vi "CSM - Message Console.vi"() -> ()   [LabVIEW 2017]
doc: "CSM Debug Console, you can use this tool:\n\n1. Select an existing CSM instance, open the front panel and block diagram.\n2. Scan the API interfaces of existing CSM instances.\n3. Select an API interface, call synchronously or asynchronously, view the return value.\n4. View the overall program's running log."
uses:
  _Support/Typedef/_CSM_GlobalLog_MSG.ctl
  _Support/Typedef/_CSM_Response Source Message.ctl
  _Support/Typedef/_CSM_GlobalLog_MSG_TYPE.ctl
  _jksm/_action.ctl
  1437127e-efa5-494e-aa43-da9d647a7a6f.vi
  6c6a0a0d-4e90-432b-9646-7a8ac0ceadb8.vi
  <vilib>/addons/_JKI Toolkits/State Machine/_JKI_lib_State_Machine.llb/Parse State Queue__JKI_lib_State_Machine.vi
  AdvanceAPI/CSM - Convert Error to Argument.vi
  _Support/GlobalEvent/GEvt-Generate with Rule Check.vi
  AdvanceAPI/CSM - Keywords.vi
  _Support/GlobalEvent/Cache-GEvt Refs.vi
  _Support/GlobalEvent/LogFilter/LogFilter - Check.vi
  <vilib>/Utility/Data Type/Get Type Information.vi
  _csmHelper/lvcsmFile/lvcsm File Path.vi
  <vilib>/Utility/config.llb/Open Config Data.vi
  <vilib>/Utility/config.llb/Read Key.vi
  <vilib>/Utility/config.llb/Read Key (Boolean).vi
  <vilib>/Utility/config.llb/Read Key (String).vi
  <vilib>/Utility/Data Type/Get Array Information.vi
  <vilib>/Utility/config.llb/Get Key Names.vi
  _csmHelper/lvcsmFile/Path to lvcsm String.vi
  _csmHelper/lvcsmFile/lvcsm String to Path.vi
  <vilib>/Utility/config.llb/Read Key (I32).vi
  <vilib>/Utility/config.llb/Read Key (Double).vi
  <vilib>/Utility/config.llb/Close Config Data.vi
  _csmHelper/lvcsmFile/_Array of VData to VCluster.vi
  <vilib>/Utility/config.llb/Write Key.vi
  <vilib>/Utility/config.llb/Write Key (Boolean).vi
  <vilib>/Utility/config.llb/Remove Key.vi
  <vilib>/Utility/config.llb/Write Key (String).vi
  <vilib>/Utility/config.llb/Write Key (I32).vi
  <vilib>/Utility/config.llb/Write Key (Double).vi
  _Polymophic/Build Synchronous Message with Arguments.vi
  _Polymophic/Build No-Reply Asynchronous Message with Arguments.vi
  _Polymophic/Build Interrupt Broadcast Message.vi
  _Support/GlobalEvent/LogFilter/LogFilter.lvclass
  Communicable State Machine.lvlib
  _csmHelper/API with lvcsm Support/CSM-Helper API with lvcsm Support.lvlib
  _csmHelper/CSM-Helper.lvclass
  _Shared/CSM Shared.lvlib
  _ui/csm-ui-support.lvlib
  _jksm/_jkism_magic.lvlib
panel:
  in  "Timeout(s)":i32=10 caption="(s)" min=1 max=180 step=1 format="%.0p"
  in  "Interface-Filter":enum16{"API-Only", "UserDef States", "All"}(ring)
  in  "Refresh API":bool
  in  "MsgString":string(combo)
  in  "Sync (-@)":bool
  in  "Async (->|)":bool
  in  "CSM":string
  in  "Arguments":string
  in  "Revert Safe String":bool=TRUE
  out "Response":string
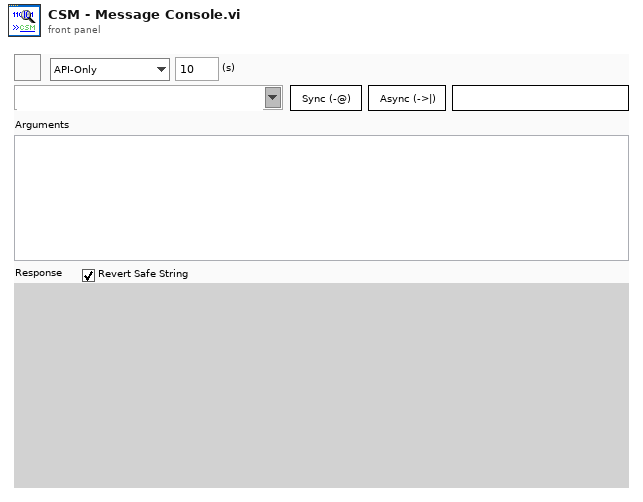
[diagram p1: front panel]
types:
  T1 = enum32{"Invalid", "Standard", "Closed", "Hidden", "Minimized", "Maximized"}
  T2 = enum32{"invalid app kind", "Development System", "Run Time System", "Student Edition", "Embedded LabVIEW", "Evaluation", "Custom"}
  T3 = cluster{"Response Timeout(s)":i32, "History Length":i32, "History":string[], "Periodic Enable":bool, "Periodic threashold(#/s)":dbl, "Periodic Check Peroid(s)":dbl}
  T4 = typedef "_jkism_magic.lvlib/_action.ctl" = enum16{"Obtain", "Destroy", "Broadcast", "Post"}
  T5 = cluster{"Shift":bool, "Ctrl":bool, "Alt":bool, "Cmd":bool, "Opt":bool}
  T6 = cluster{"Core":cluster{"Current VI Reference":refnum<vi>, "Close Panel on Exit?":bool}, "CSM Global Log Event":refnum<user-event>, "Toobar.advance":refnum<vi>[], "CSM Check History":string[], "History Length":i32}
  T7 = cluster{"Current VI Reference":refnum<vi>, "Close Panel on Exit?":bool}
  T8 = enum8{"Enabled", "Disabled", "Disabled and Grayed Out"}
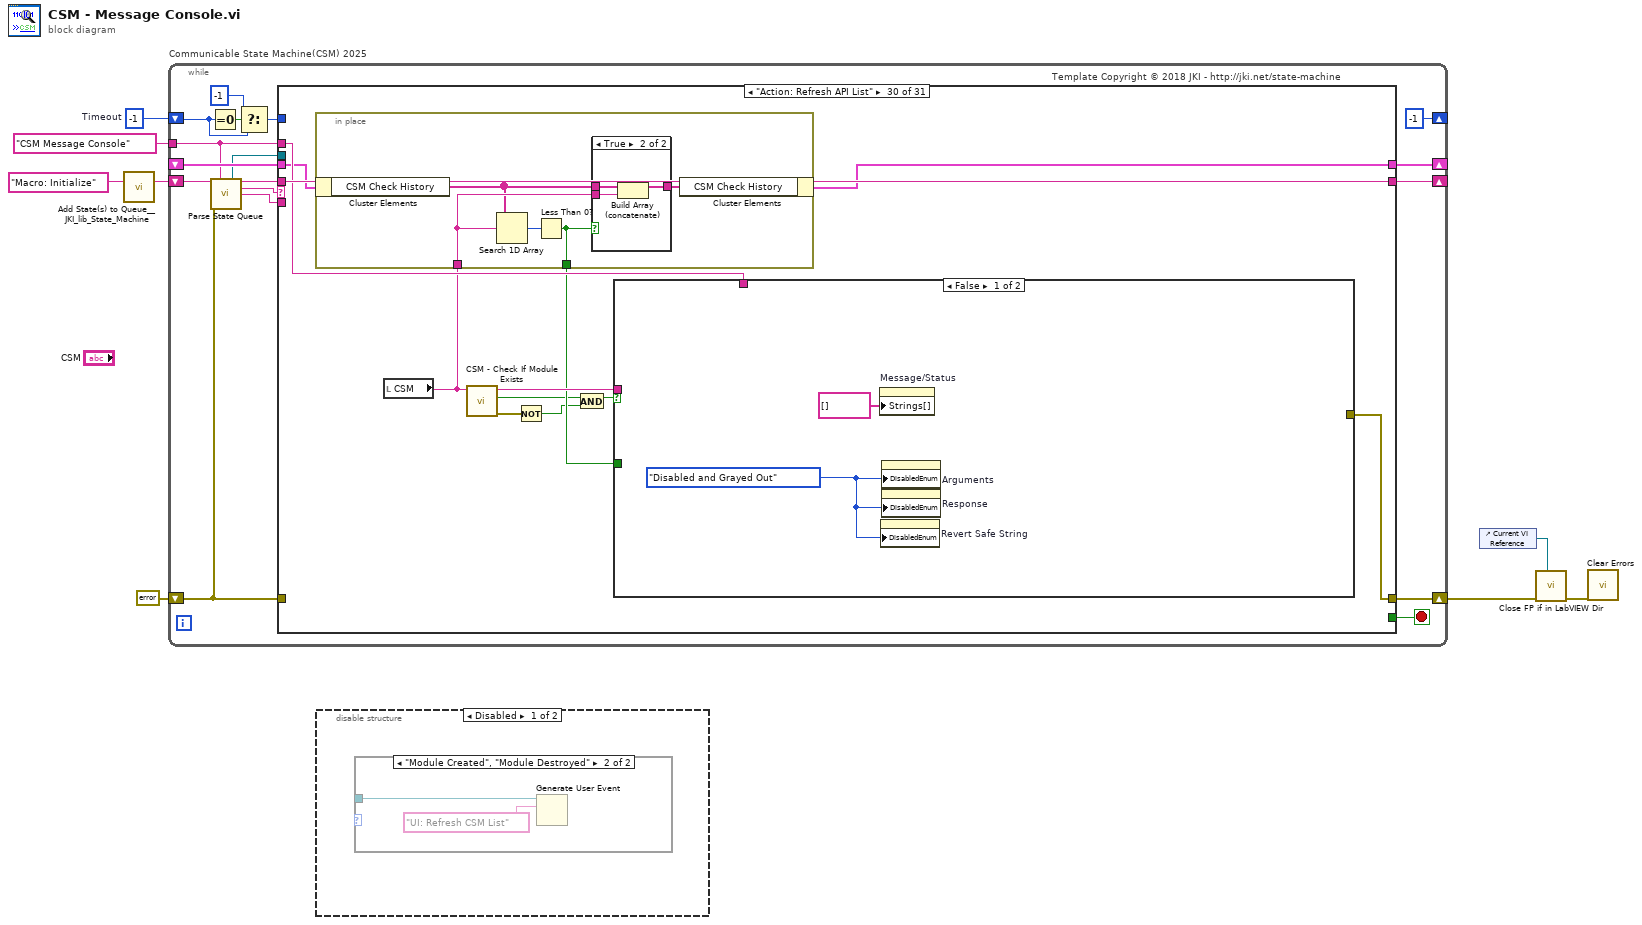
[diagram p0: block diagram]
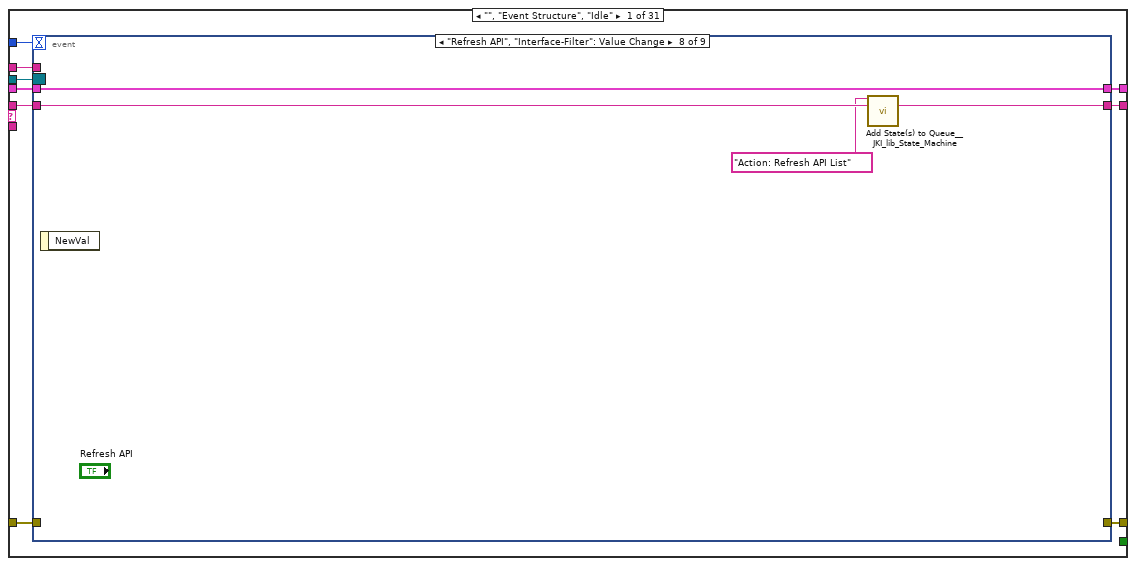
[diagram p4: hidden frame]
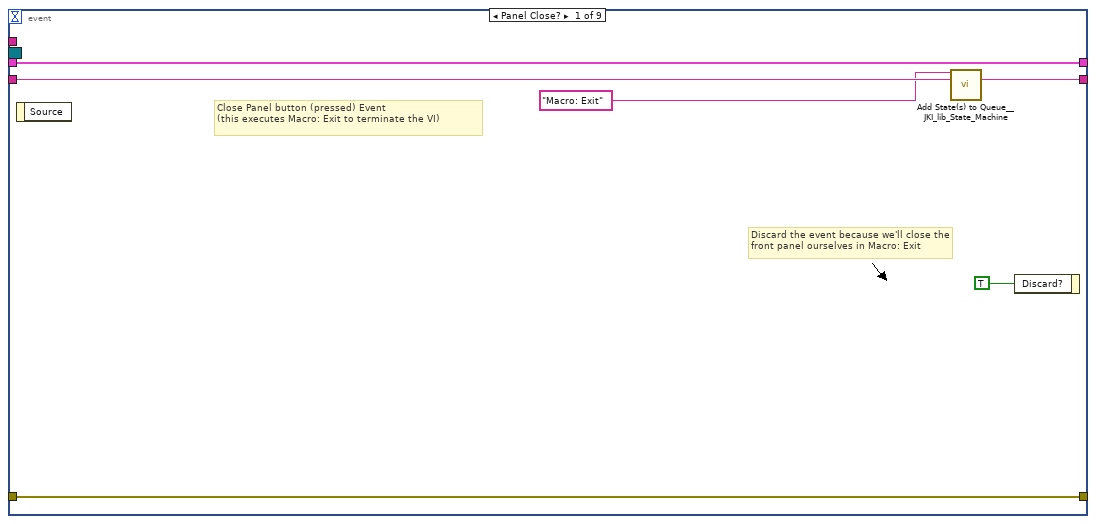
[diagram p5: hidden frame]
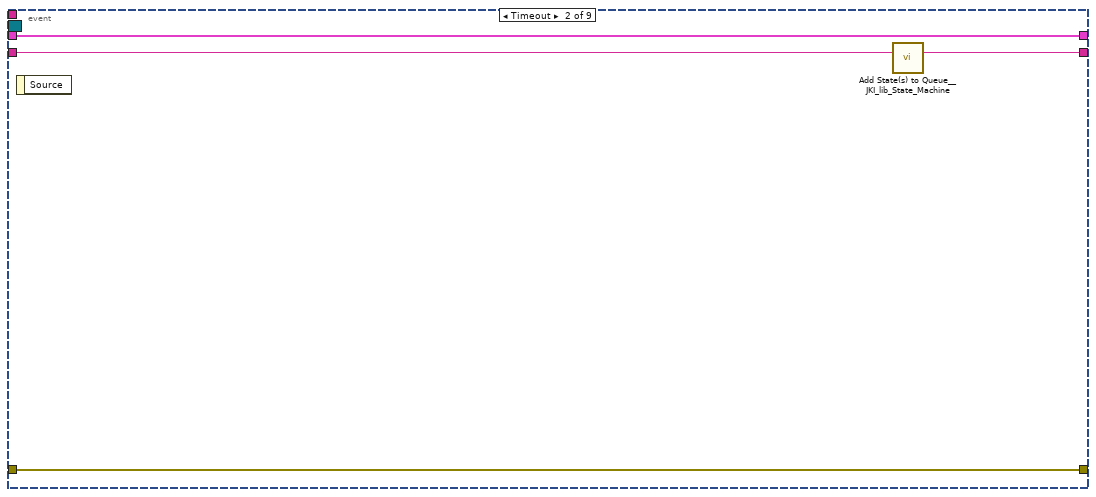
[diagram p6: hidden frame]
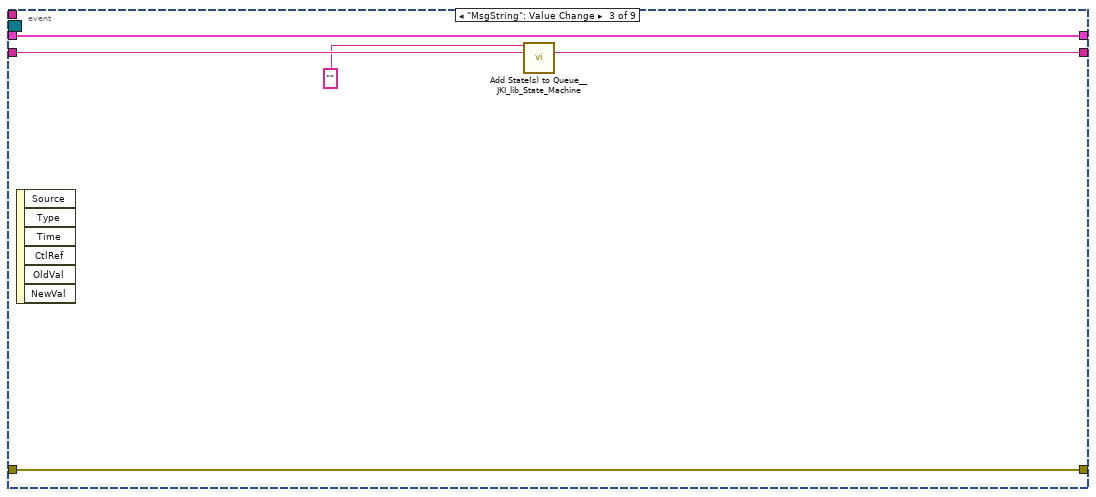
[diagram p7: hidden frame]
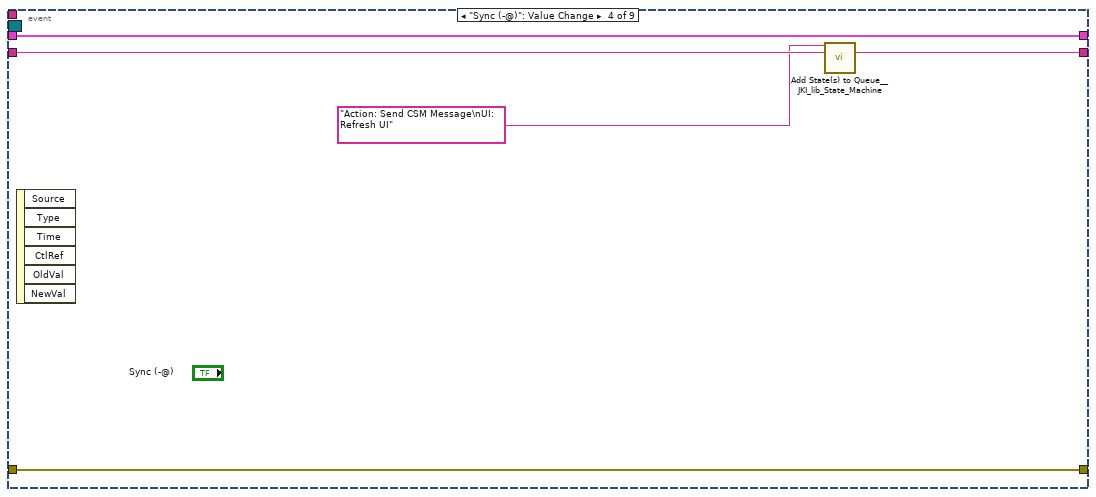
[diagram p8: hidden frame]
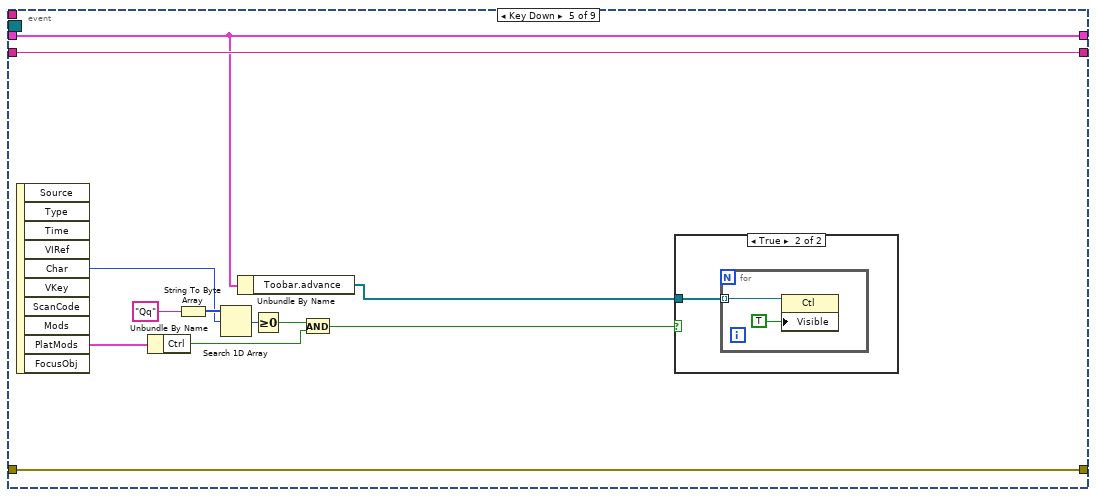
[diagram p9: hidden frame]
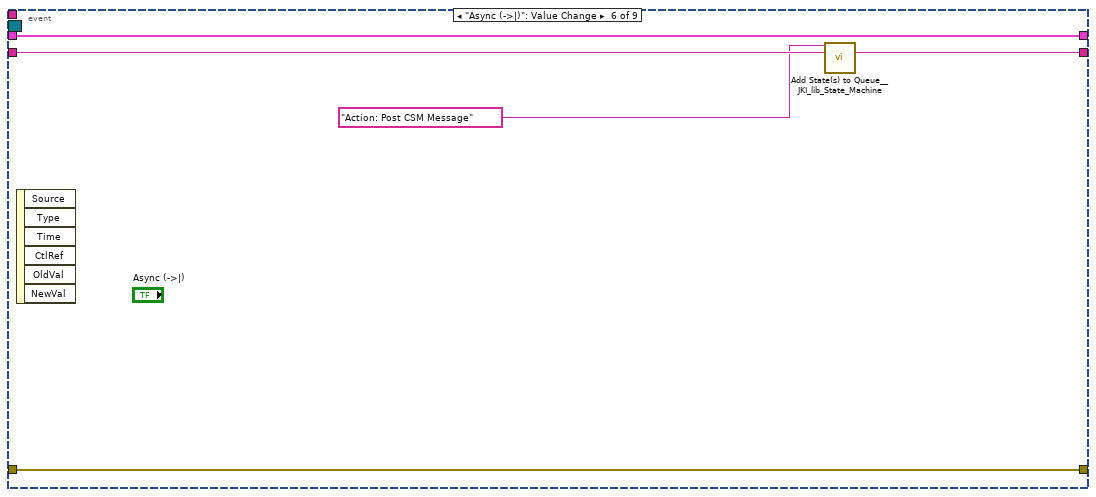
[diagram p11: hidden frame]
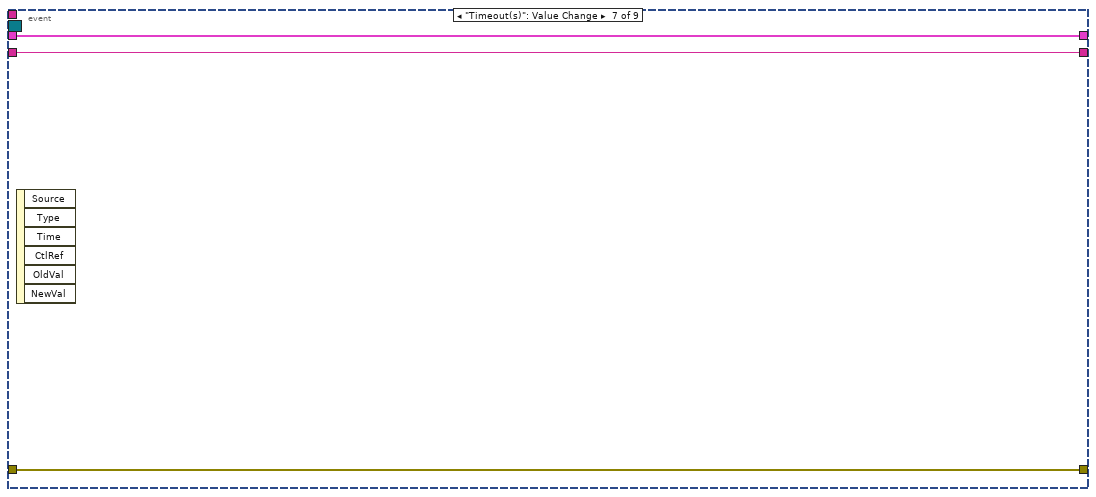
[diagram p12: hidden frame]
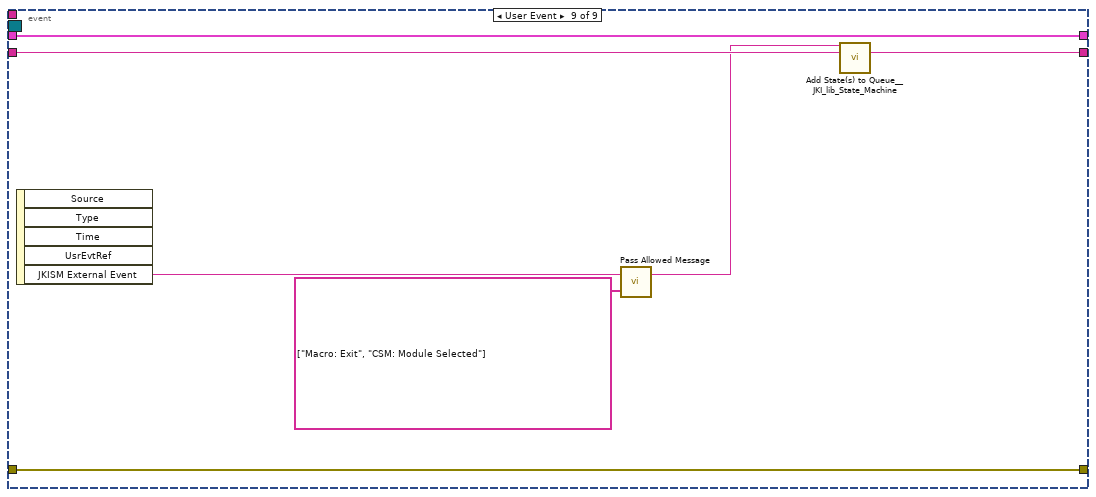
[diagram p13: hidden frame]
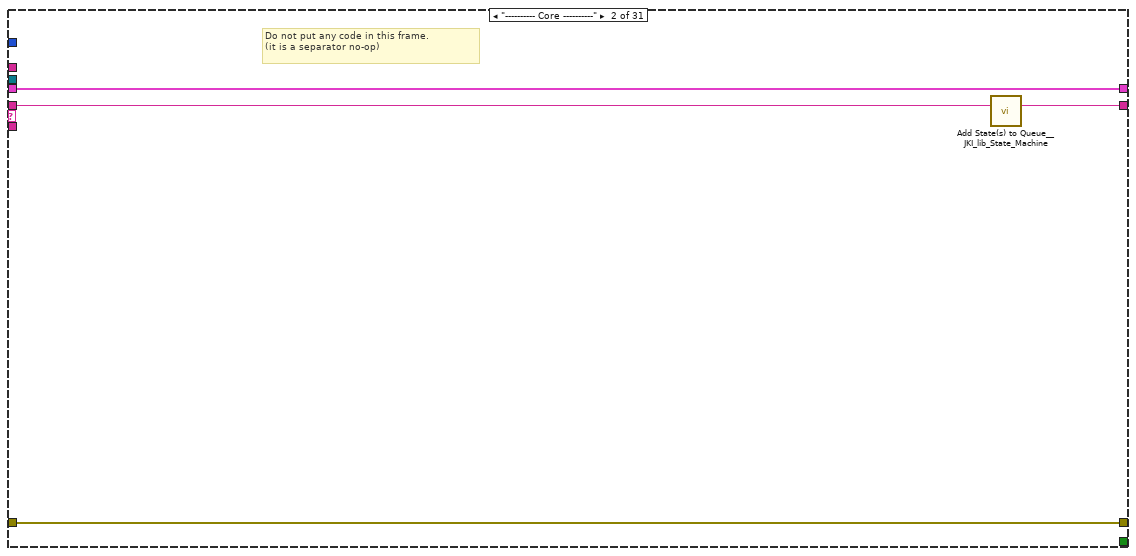
[diagram p14: hidden frame]
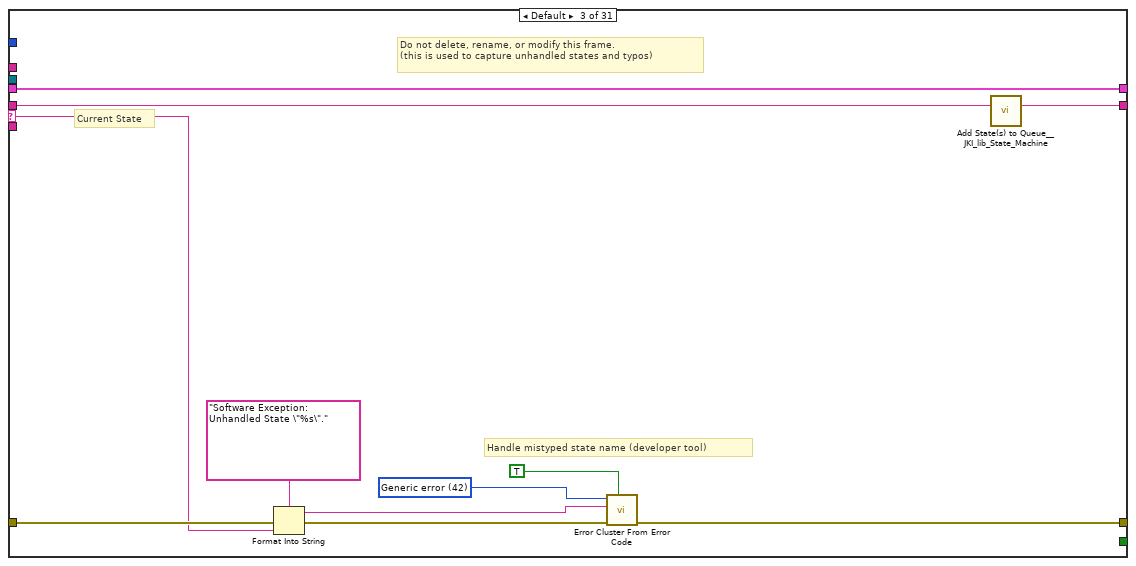
[diagram p15: hidden frame]
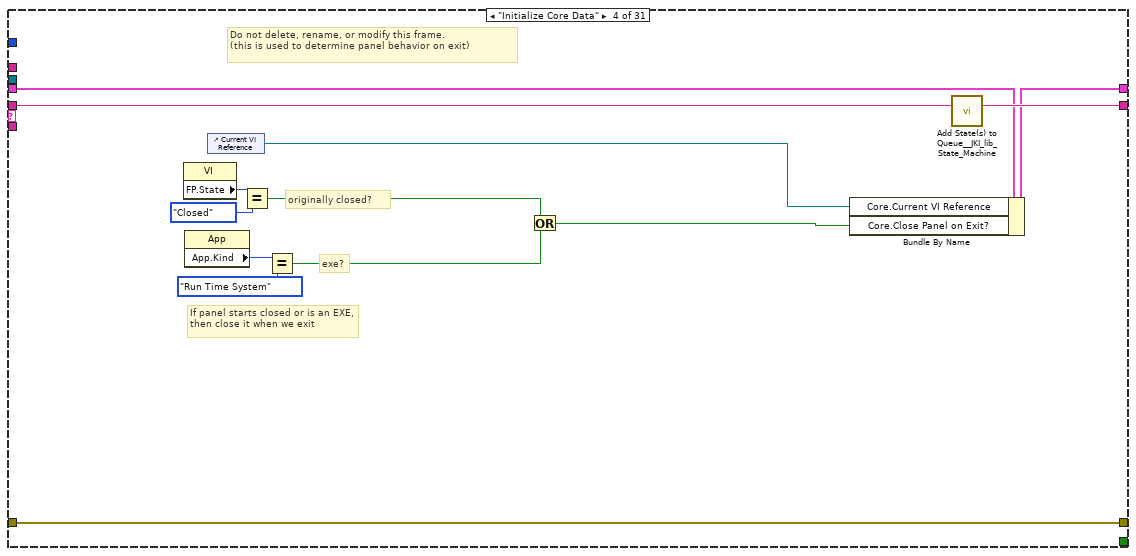
[diagram p16: hidden frame]
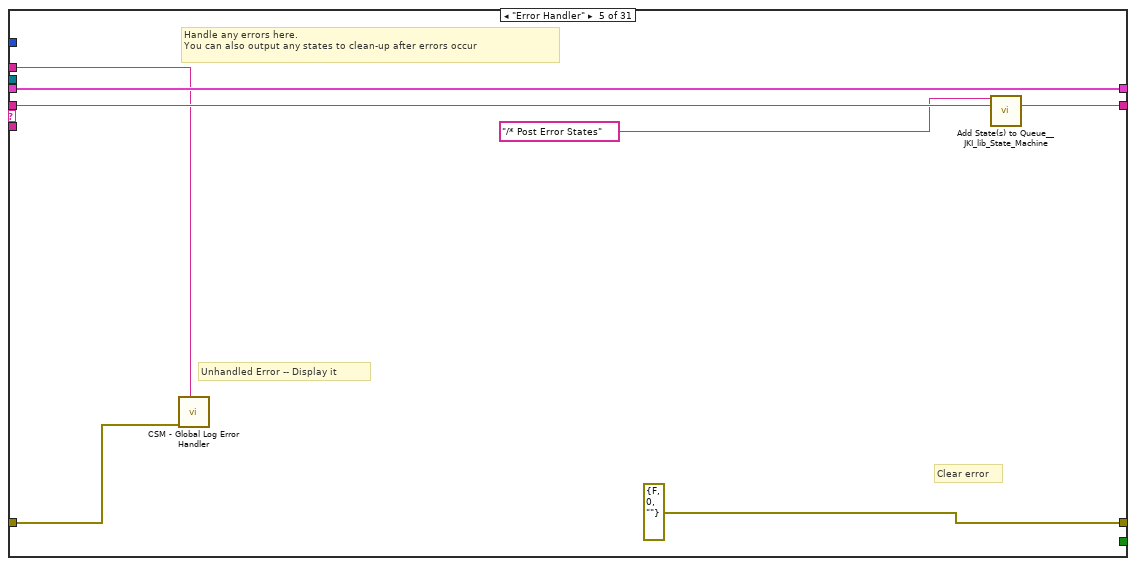
[diagram p17: hidden frame]
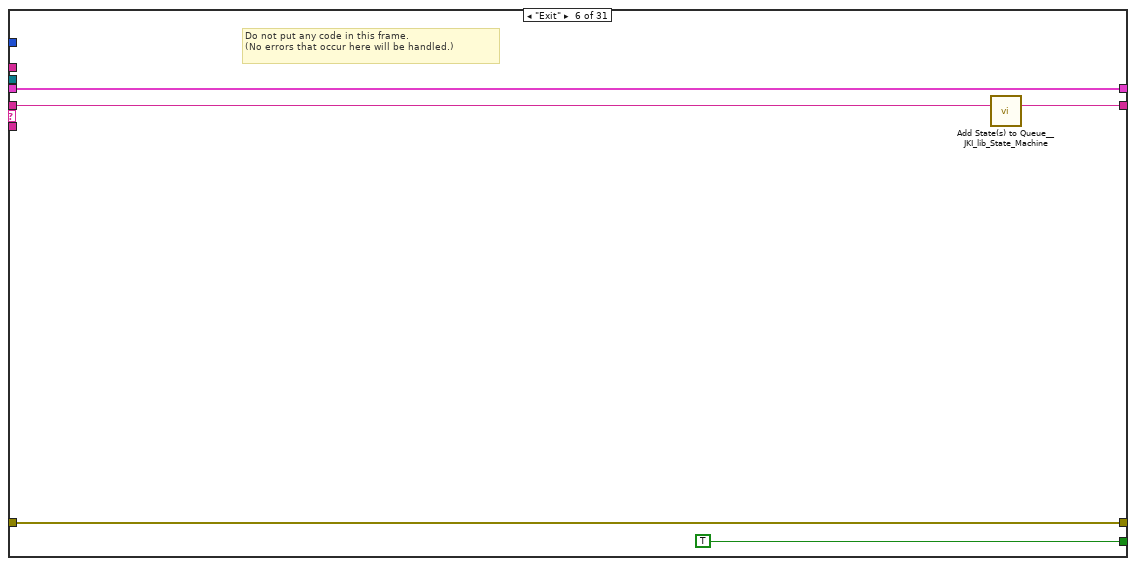
[diagram p18: hidden frame]
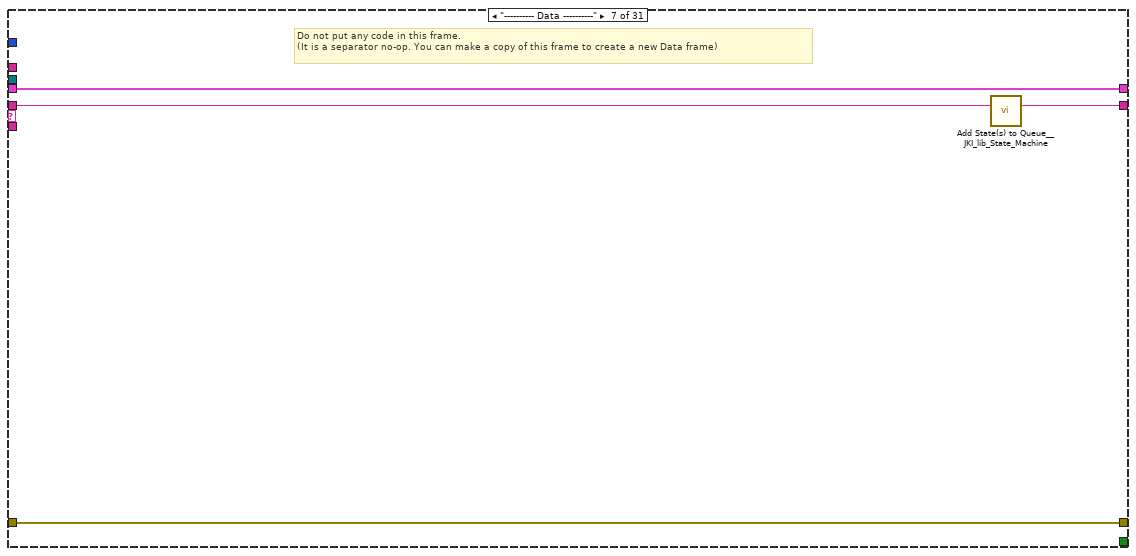
[diagram p19: hidden frame]
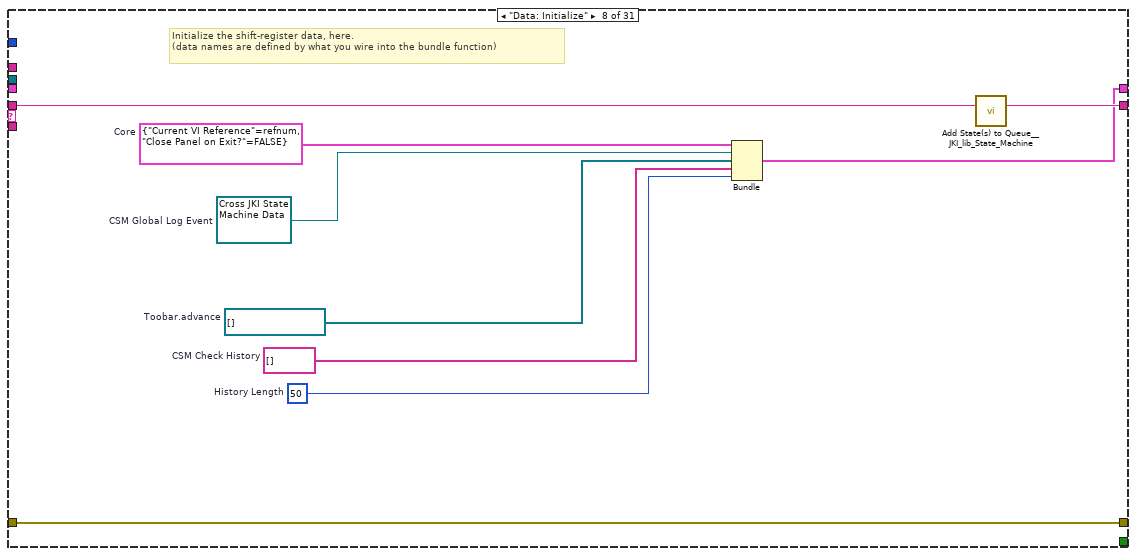
[diagram p20: hidden frame]
diagram:
  w6 = -1  # Timeout
  n1 = call <vilib>:"Add State(s) to Queue__JKI_lib_State_Machine.vi"("State(s) in (\"\")"="Macro: Initialize") -> ("States Out"=w7:string)  [unwired: 14 in]
  n2 = while "Communicable State Machine(CSM) 2025" {
    shift-right: [w18] -> _
    shift-left: _ -> [w17]
    shift-right: [w21] -> w3
    shift-left: errorcluster {"status"=FALSE, "code"=0, "source"=""} ("error out") -> [w16]
    shift-right: [w20] -> _
    shift-left: w7 -> [w22]
    tunnel: "CSM Message Console" -> [w10]
    shift-right: [-1 ("Timeout")] -> _
    shift-left: w6 -> [w13]
    stop <- w19 stop-if-true
    # "Template Copyright © 2018 JKI - http://jki.net/state-machine"
    n3 = Equal To 0?(x=w13) -> (x = 0?=w15:bool)
    n4 = call "Parse State Queue.vi"("State Queue"=w22, "Current Module(\"\" to generate an ID)"=w10, "Error In (no error)"=w16) -> ("Event Registration Refnum"=w9:refnum<event-registration>, "Remaining States"=w24:string, "Current State"=w25:string, "Arguments"=w23:string)  [unwired: 9 in]
    n5 = Select(t=-1 ("Timeout"), s=w15, f=w13) -> (s? t:f=w12:i32)
    n6 = case shown="\"Action: Refresh API List\"" w25 {
      selector: w25 -> [_ _ w93 _ _ _ _ _ _ _ _ _ _ _ _ _ _ _ _ _ _ _ _ _ _ _ _ _ _ _ _]
      tunnel: w24 -> [w34 w92 w97 w116 w123 w128 w132 w141 w143 w152 w160 w166 w170 w174 w181 w190 w201 w276 w283 w286 w292 w297 w302 w310 w314 w325 w350 w369 w383 w396 w424]
      tunnel: w23 -> [_ _ _ _ _ _ _ _ _ _ _ _ _ _ _ w185 w195 w275 _ w288 _ _ _ _ _ _ _ _ _ _ _]
      tunnel: w17 -> [w32 w89 w95 w109 w120 w126 w129 _ w142 w150 w159 w161 w167 w171 w178 w188 w197 w273 w282 w289 w291 w294 w299 w307 w311 w323 w348 w367 w382 w391 w423]
      tunnel: [w31 w90 w99 w113 errorcluster {"status"=FALSE, "code"=0, "source"=""} ("error out") w125 w130 w138 w144 _ w155 w162 w168 w172 w179 w186 w198 w277 w284 w290 w293 w295 w300 w308 w312 w320 w347 w366 w384 w393 w425] -> w21
      tunnel: w16 -> [w30 w90 w98 w113 w119 w125 w130 w138 w144 _ _ w163 w168 w172 w179 w187 w199 w277 w284 w290 w293 w295 w300 w308 w312 _ _ _ w384 _ w425]
      tunnel: [w33 w91 w96 w115 w122 w127 w131 w140 w143 w152 w160 w165 w169 w173 w180 w189 w200 w276 w283 w287 w292 w296 w301 w309 w313 w324 w349 w368 w383 w396 w424] -> w20
      tunnel: [_ _ _ _ _ TRUE _ _ _ _ _ _ _ _ _ _ _ _ _ _ _ _ _ _ _ _ _ _ _ _ _] -> w19
      tunnel: [w29 w89 w95 w114 w120 w126 w129 w139 w142 w151 w159 w161 w167 w171 w178 w188 w197 w273 w282 w289 w291 w294 w299 w307 w311 w323 w348 w367 w382 w390 w423] -> w18
      tunnel: w12 -> [w28 _ _ _ _ _ _ _ _ _ _ _ _ _ _ _ _ _ _ _ _ _ _ _ _ _ _ _ _ _ _]
      tunnel: w10 -> [w27 _ _ _ w117 _ _ _ _ w147 w156 _ _ _ _ _ _ _ _ _ _ _ _ _ _ _ _ _ _ w394 _]
      tunnel: w9 -> [w26 _ _ _ _ _ _ _ _ _ _ _ _ _ _ _ _ _ _ _ _ _ _ _ _ _ _ _ _ _ _]
      frame "", "Event Structure", "Idle" {
        n7 = event shown="[7] \"Refresh API\", \"Interface-Filter\": Value Change" {
          selector: w26 -> [_ _ _ _ _ _ _ _ _]
          dyn-events: _ -> [_ _ _ _ _ _ _ _ _]
          timeout: w28 -> [_ _ _ _ _ _ _ _ _]
          tunnel: w34 -> [w40 w44 w46 w51 w66 w71 w77 w79 w85]
          tunnel: [w39 w43 w47 w52 w66 w72 w77 w80 w86] -> w33
          tunnel: w32 -> [w37 w41 w48 w53 w55 w73 w75 w81 w87]
          tunnel: [w38 w42 w49 w54 w65 w74 w76 _ w88] -> w31
          tunnel: w30 -> [w38 w42 w49 w54 w65 w74 w76 _ w88]
          tunnel: [w37 w41 w48 w53 w55 w73 w75 w81 w87] -> w29
          tunnel: w27 -> [_ _ _ _ _ _ _ _ _]
          event Panel Close? {
            # "Discard the event because we'll close the front panel ourselves in Macro: Exit"
            # "Close Panel button (pressed) Event\n(this executes Macro: Exit to terminate the VI)"
            n8 = event-data() -> ()  [unwired: 1 in, 1 out]
            n9 = call <vilib>:"Add State(s) to Queue__JKI_lib_State_Machine.vi"("State(s) in Front (\"\")"="Macro: Exit", "State(s) in (\"\")"=w40) -> ("States Out"=w39:string)  [unwired: 13 in]
            n10 = event-data("Discard?"=TRUE) -> ()  [unwired: 1 in, 1 out]
          }
          event Timeout {
            n11 = event-data() -> ()  [unwired: 1 in, 1 out]
            n12 = call <vilib>:"Add State(s) to Queue__JKI_lib_State_Machine.vi"("State(s) in (\"\")"=w44) -> ("States Out"=w43:string)  [unwired: 14 in]
          }
          event "MsgString": Value Change {
            n13 = event-data() -> ()  [unwired: 1 in, 6 out]
            n14 = call <vilib>:"Add State(s) to Queue__JKI_lib_State_Machine.vi"("State(s) in Front (\"\")"="" ("State(s) in Front (\"\")"), "State(s) in (\"\")"=w46) -> ("States Out"=w47:string)  [unwired: 13 in]
          }
          event "Sync (-@)": Value Change {
            n15 = event-data() -> ()  [unwired: 1 in, 6 out]
            n16 = call <vilib>:"Add State(s) to Queue__JKI_lib_State_Machine.vi"("State(s) in Front (\"\")"="Action: Send CSM Message\nUI: Refresh UI" ("State(s) in Front (\"\")"), "State(s) in (\"\")"=w51) -> ("States Out"=w52:string)  [unwired: 13 in]
          }
          event Key Down {
            n17 = event-data() -> ("Char"=w56:i16, "PlatMods"=w57:T5)  [unwired: 1 in, 8 out]
            n18 = Unbundle By Name(w57) -> ("Ctrl"=w60:bool)
            n19 = String To Byte Array(string="Qq") -> (unsigned byte array=w62:u8[])
            n20 = Search 1D Array(1D array=w62, element=w56) -> (index of element=w63:i32)  [unwired: 1 in]
            n21 = Unbundle By Name(w55) -> ("Toobar.advance"=w58:refnum<vi>[])
            n22 = Greater Or Equal To 0?(x=w63) -> (x >= 0?=w64:bool)
            n23 = And(x=w64, y=w60) -> (x .and. y?=w59:bool)
            n24 = case shown="True" w59 {
              tunnel: w58 -> [_ w67]
              frame False {
              }
              frame True {
                n25 = for {
                  tunnel: w67 -> [w69] mode=indexing
                  n26 = property class="Ctl"(reference=w69, "Visible"=TRUE) -> ()  [unwired: 1 in, 2 out]
                }
              }
            }
          }
          event "Async (->|)": Value Change {
            n27 = event-data() -> ()  [unwired: 1 in, 6 out]
            n28 = call <vilib>:"Add State(s) to Queue__JKI_lib_State_Machine.vi"("State(s) in Front (\"\")"="Action: Post CSM Message" ("State(s) in Front (\"\")"), "State(s) in (\"\")"=w71) -> ("States Out"=w72:string)  [unwired: 13 in]
          }
          event "Timeout(s)": Value Change {
            n29 = event-data() -> ()  [unwired: 1 in, 6 out]
          }
          event "Refresh API", "Interface-Filter": Value Change {
            n30 = event-data() -> ()  [unwired: 1 in, 1 out]
            n31 = call <vilib>:"Add State(s) to Queue__JKI_lib_State_Machine.vi"("State(s) in Front (\"\")"="Action: Refresh API List" ("State(s) in Front (\"\")"), "State(s) in (\"\")"=w79) -> ("States Out"=w80:string)  [unwired: 13 in]
          }
          event User Event {
            n32 = event-data() -> ("JKISM External Event"=w84:string)  [unwired: 1 in, 4 out]
            n33 = call "Pass Allowed Message.vi"("Allowed Message"=string[] ["Macro: Exit", "CSM: Module Selected"], "JKISM External Event"=w84) -> ("States"=w83:string)  [unwired: 1 in]
            n34 = call <vilib>:"Add State(s) to Queue__JKI_lib_State_Machine.vi"("State(s) in Front (\"\")"=w83, "State(s) in (\"\")"=w85) -> ("States Out"=w86:string)  [unwired: 13 in]
          }
        }
      }
      frame "---------- Core ----------" {
        # "Do not put any code in this frame.\n(it is a separator no-op)"
        n35 = call <vilib>:"Add State(s) to Queue__JKI_lib_State_Machine.vi"("State(s) in (\"\")"=w92) -> ("States Out"=w91:string)  [unwired: 14 in]
      }
      frame Default {
        w102 = 42 items=["No error", "Argument error", "Memory is full", "Out of zone", "End of file", "File already open", "Generic file I/O error", "File not found", "File permission error", "Disk is full", "Duplicate path", "Too many files open", "System feature not enabled", "Resource file not found", "Cannot add resource", "Resource not found", "Image not found", "Image memory error", "Pen does not exist", "Config type invalid", "Config token not found", "Config parse error", "Config memory error", "Bad external code format", "Bad external code offset", "External code not present", "Null window", "Destroy window error", "Null menu", "Print aborted", "Bad print record", "Print driver error", "Windows error during printing", "Memory error during printing", "Print dialog error", "Generic print error", "Invalid device refnum", "Device not found", "Device parameter error", "Device unit error", "Cannot open device", "Device call aborted", "Generic error", "Cancelled by user", "Object ID too low", "Object ID too high", "Object not in heap", "Unknown heap", "Unknown object (invalid DefProc)", "Unknown object (DefProc not in table)", "Message out of range", "Invalid (null) method", "Unknown message", "Manager call not supported", "Bad address", "Network operation in progress", "Network operation timed out", "Connection is busy", "Network attribute not supported", "Network error", "Address in use", "System out of memory", "Connection aborted", "Connection refused", "Not connected", "Already connected", "Connection closed", "Initialization error (interapplication manager)", "Bad occurrence", "Wait on unbound occurrence handler", "Occurrence queue overflow", "Datalog type conflict", "Unused", "Unrecognized type (interapplication manager)", "Memory corrupt", "Failed to make temporary DLL", "Old CIN version", "Drag socket not found", "Failed to load drop-object", "Failed to register OLE object", "Failed to release OLE object", "Format specifier type mismatch", "Unknown format specifier", "Too few format specifiers", "Too many format specifiers", "Scan failed", "Newer CIN version", "Error converting to variant", "Runtime menu error", "Password tampered", "Variant attribute not found", "Incompatible variant data type", "Event data is not available", "Event Store is not present", "Occurrence is not found", "Event Queue is not created", "Event info is not available", "Refnum passed is NULL", "Error retrieving Class GUID", "Error retrieving CoClass GUID", "Error retrieving TypeLib GUID.", "Bad built application magic bytes.", "Specific driver is different from the specific driver associated with the Logical Name.", "There is no session opened to the class driver.", "Max Error", "MAX - Error with config objects", "MAX - Error loading configuration", "MAX - Group not supported"]
        # "Current State"
        # "Do not delete, rename, or modify this frame.\n(this is used to capture unhandled states and typos)"
        # "Handle mistyped state name (developer tool)"
        n36 = Format Into String(format string="Software Exception: Unhandled State \"%s\"." ("message"), error in=w98, w93) -> (resulting string=w101:string, error out=w100:errorcluster)  [unwired: 1 in]
        n37 = call <vilib>:"Error Cluster From Error Code.vi"("show call chain? (False)"=TRUE, "error in (no error)"=w100, "error message (\"\")"=w101, "error code (0)"=w102) -> ("error out"=w99:errorcluster)  [unwired: 5 in]
        n38 = call <vilib>:"Add State(s) to Queue__JKI_lib_State_Machine.vi"("State(s) in (\"\")"=w97) -> ("States Out"=w96:string)  [unwired: 14 in]
      }
      frame "Initialize Core Data" {
        # "Do not delete, rename, or modify this frame.\n(this is used to determine panel behavior on exit)"
        # "originally closed?"
        # "exe?"
        # "If panel starts closed or is an EXE, then close it when we exit"
        n39 = property class="VI"() -> ("FP.State"=w106:T1)  [unwired: 2 in, 2 out]
        n40 = property class="App"() -> ("App.Kind"=w112:T2)  [unwired: 2 in, 2 out]
        n41 = control-ref of="Current VI Reference"() -> (w107:refnum<vi>)
        n42 = Equal?(x=w106, y=T1."Closed" ("Front Panel Window:State")) -> (x = y?=w104:bool)
        n43 = Equal?(x=w112, y=T2."Run Time System" ("Application:Kind")) -> (x = y?=w110:bool)
        n44 = Or(x=w104, y=w110) -> (x .or. y?=w108:bool)
        n45 = Bundle By Name(cluster=w109, "Core.Current VI Reference"=w107, "Core.Close Panel on Exit?"=w108) -> (w114:T6)
        n46 = call <vilib>:"Add State(s) to Queue__JKI_lib_State_Machine.vi"("State(s) in (\"\")"=w116) -> ("States Out"=w115:string)  [unwired: 14 in]
      }
      frame "Error Handler" {
        # "Unhandled Error -- Display it"
        # "Handle any errors here.\nYou can also output any states to clean-up after errors occur"
        # "Clear error"
        n47 = call "CSM - Global Log Error Handler.vi"("Place (\"\" to Use VI's Name)"=w117, "Error In"=w119) -> ()  [unwired: 9 in, 1 out]
        n48 = call <vilib>:"Add State(s) to Queue__JKI_lib_State_Machine.vi"("State(s) in Front (\"\")"="/* Post Error States", "State(s) in (\"\")"=w123) -> ("States Out"=w122:string)  [unwired: 13 in]
      }
      frame "Exit" {
        # "Do not put any code in this frame.\n(No errors that occur here will be handled.)"
        n49 = call <vilib>:"Add State(s) to Queue__JKI_lib_State_Machine.vi"("State(s) in (\"\")"=w128) -> ("States Out"=w127:string)  [unwired: 14 in]
      }
      frame "---------- Data ----------" {
        # "Do not put any code in this frame.\n(It is a separator no-op. You can make a copy of this frame to create a new Data frame)"
        n50 = call <vilib>:"Add State(s) to Queue__JKI_lib_State_Machine.vi"("State(s) in (\"\")"=w132) -> ("States Out"=w131:string)  [unwired: 14 in]
      }
      frame "Data: Initialize" {
        w133 = 50  # History Length
        w134 = string[] []  # CSM Check History
        w135 = refnum<vi>[] []  # Toobar.advance
        w136 = refnum<user-event> refnum  # CSM Global Log Event
        w137 = T7 {"Current VI Reference"=refnum, "Close Panel on Exit?"=FALSE}  # Core
        # "Initialize the shift-register data, here.\n(data names are defined by what you wire into the bundle function)"
        n51 = Bundle("Core"=w137, "CSM Global Log Event"=w136, "Toobar.advance"=w135, "CSM Check History"=w134, "History Length"=w133) -> (w139:T6)  [unwired: 1 in]
        n52 = call <vilib>:"Add State(s) to Queue__JKI_lib_State_Machine.vi"("State(s) in (\"\")"=w141) -> ("States Out"=w140:string)  [unwired: 14 in]
      }
      frame "Data: Initialize References" {
      }
      frame "Data: Load Arguments Config File" {
        n53 = call "lvcsm Read Cluster.vim"("Section"=w147, "Default Prototype"=T3 {"Response Timeout(s)"=30, "History Length"=50, "History"=[], "Periodic Enable"=TRUE, "Periodic threashold(#/s)"=0.5, "Periodic Check Peroid(s)"=3.0}) -> ("Cluster (Dup)"=w149:T3)  [unwired: 8 in, 1 out]
        n54 = Unbundle By Name(w149) -> ("Response Timeout(s)"=w148:i32, "History Length"=w145:i32)  [unwired: 4 out]
        n55 = local write "Timeout(s)"(w148) -> ()
        n56 = Bundle By Name(cluster=w150, "History Length"=w145) -> (w151:T6)
      }
      frame "Data: Save Arguments Config File" {
        n57 = Unbundle By Name(w159) -> ("History Length"=w153:i32)
        n58 = local read "Timeout(s)"() -> (w157:i32)
        n59 = Bundle By Name(cluster=T3 {"Response Timeout(s)"=30, "History Length"=50, "History"=[], "Periodic Enable"=TRUE, "Periodic threashold(#/s)"=0.5, "Periodic Check Peroid(s)"=3.0}, "Response Timeout(s)"=w157, "History Length"=w153) -> (w158:T3)
        n60 = call "lvcsm Write Cluster.vim"("Section"=w156, "Configuration"=w158) -> ("error out"=w155:errorcluster)  [unwired: 9 in]
      }
      frame "Data: Cleanup" {
        # "Cleanup any data and references, here.\n(this is called automatically, by the Macro: Exit)"
        n61 = Unbundle By Name(w161) -> ("Core.Current VI Reference"=w164:refnum<vi>)
        n62 = Close Reference(reference=w164, error in (no error)=w163) -> (error out=w162:errorcluster)
        n63 = call <vilib>:"Add State(s) to Queue__JKI_lib_State_Machine.vi"("State(s) in (\"\")"=w166) -> ("States Out"=w165:string)  [unwired: 14 in]
      }
      frame "---------- Events ----------" {
        # "Do not put any code in this frame.\n(It is a separator no-op. You can make a copy of this frame to create a new UI frame)"
        n64 = call <vilib>:"Add State(s) to Queue__JKI_lib_State_Machine.vi"("State(s) in (\"\")"=w170) -> ("States Out"=w169:string)  [unwired: 14 in]
      }
      frame "---------- UI ----------" {
        # "Do not put any code in this frame.\n(It is a separator no-op. You can make a copy of this frame to create a new UI frame)"
        n65 = call <vilib>:"Add State(s) to Queue__JKI_lib_State_Machine.vi"("State(s) in (\"\")"=w174) -> ("States Out"=w173:string)  [unwired: 14 in]
      }
      frame "UI: Initialize" {
        # "Initialize the User Interface, here.\n(this is called automatically, by the Macro: Init)"
        n66 = Unbundle By Name(w178) -> ("Toobar.advance"=w177:refnum<vi>[])
        n67 = disable-structure shown="Disabled" {
          disable-tunnel: w177 -> [w182 _]
          frame Disabled {
            n68 = for {
              tunnel: w182 -> [w184] mode=indexing
              n69 = property class="Ctl"(reference=w184, "Visible"=FALSE) -> ()  [unwired: 1 in, 2 out]
            }
          }
          frame Enabled {
          }
        }
        n70 = local write "Response"(" " ("State History")) -> ()
        n71 = local write "Interface-Filter"(enum16{"API-Only", "UserDef States", "All"}."UserDef States" ("Interface-Filter")) -> ()
        n72 = call <vilib>:"Add State(s) to Queue__JKI_lib_State_Machine.vi"("State(s) in (\"\")"=w181) -> ("States Out"=w180:string)  [unwired: 14 in]
      }
      frame "UI: Cursor Set" {
        # "Argument"
        # "Set and Unset Cursor Busy.\n(Usage: \"UI: Cursor Set >> Busy|Idle\")"
        n73 = case shown="\"Idle\", Default" w185 {
          tunnel: w187 -> [w192 w194]
          tunnel: [w191 w193] -> w186
          frame "Idle", Default {
            n74 = call <vilib>:"Unset Busy.vi"("error in (no error)"=w192) -> ("error out"=w191:errorcluster)  [unwired: 10 in]
          }
          frame "Busy" {
            n75 = call <vilib>:"Set Busy.vi"("error in (no error)"=w194) -> ("error out"=w193:errorcluster)  [unwired: 9 in, 1 out]
          }
        }
        n76 = call <vilib>:"Add State(s) to Queue__JKI_lib_State_Machine.vi"("State(s) in (\"\")"=w190) -> ("States Out"=w189:string)  [unwired: 14 in]
      }
      frame "UI: Front Panel State" {
        # "Argument"
        # "Set Front Panel Open or Closed\n(Usage: \"UI: Front Panel State >> Open|Close\")"
        n77 = Unbundle By Name(w197) -> ("Core.Current VI Reference"=w196:refnum<vi>)
        n78 = case shown="\"Minimize\", \"Minimized\"" w195 {
          tunnel: w199 -> [w207 w222 w233 w246 w259]
          tunnel: [w209 w223 w235 w248 w261] -> w198
          tunnel: w196 -> [w208 w220 w234 w247 w260]
          frame "Open", "Standard", Default {
            w202 = T1."Standard" ("State")
            n79 = property class="VI"(reference=w208, error in=w207) -> (reference out=w205:refnum<vi>, error out=w206:errorcluster, "FP.State"=w204:T1)
            n80 = Not Equal?(x=w204, y=w202) -> (x != y?=w203:bool)
            n81 = case shown="True" w203 {
              tunnel: [w213 w215] -> w209
              tunnel: w206 -> [w212 w215]
              tunnel: w205 -> [w211 _]
              tunnel: w202 -> [w210 _]
              frame True {
                n82 = invoke class="VI" method="FP.Open"(reference=w211, error in=w212, "Activate"=TRUE, "State"=w210) -> (error out=w213:errorcluster)  [unwired: 1 in, 4 out]
              }
              frame False {
              }
            }
          }
          frame "Close", "Closed" {
            n83 = property class="VI"(reference=w220, error in=w222) -> (reference out=w219:refnum<vi>, error out=w221:errorcluster, "FP.State"=w217:T1)
            n84 = Not Equal?(x=w217, y=T1."Closed" ("Front Panel Window:State")) -> (x != y?=w216:bool)
            n85 = case shown="True" w216 {
              tunnel: [w224 w227] -> w223
              tunnel: w221 -> [w224 w226]
              tunnel: w219 -> [_ w225]
              frame False {
              }
              frame True {
                n86 = invoke class="VI" method="FP.Close"(reference=w225, error in=w226) -> (error out=w227:errorcluster)  [unwired: 1 in, 2 out]
              }
            }
          }
          frame "Hidden", "Hide" {
            w228 = T1."Hidden" ("State")
            n87 = property class="VI"(reference=w234, error in=w233) -> (reference out=w231:refnum<vi>, error out=w232:errorcluster, "FP.State"=w230:T1)
            n88 = Not Equal?(x=w230, y=w228) -> (x != y?=w229:bool)
            n89 = case shown="True" w229 {
              tunnel: [w239 w240] -> w235
              tunnel: w232 -> [w238 w240]
              tunnel: w231 -> [w237 _]
              tunnel: w228 -> [w236 _]
              frame True {
                n90 = invoke class="VI" method="FP.Open"(reference=w237, error in=w238, "State"=w236) -> (error out=w239:errorcluster)  [unwired: 2 in, 4 out]
              }
              frame False {
              }
            }
          }
          frame "Minimize", "Minimized" {
            w241 = T1."Minimized" ("State")
            n91 = property class="VI"(reference=w247, error in=w246) -> (reference out=w244:refnum<vi>, error out=w245:errorcluster, "FP.State"=w243:T1)
            n92 = Not Equal?(x=w243, y=w241) -> (x != y?=w242:bool)
            n93 = case shown="True" w242 {
              tunnel: [w252 w253] -> w248
              tunnel: w245 -> [w251 w253]
              tunnel: w244 -> [w250 _]
              tunnel: w241 -> [w249 _]
              frame True {
                n94 = invoke class="VI" method="FP.Open"(reference=w250, error in=w251, "State"=w249) -> (error out=w252:errorcluster)  [unwired: 2 in, 4 out]
              }
              frame False {
              }
            }
          }
          frame "Maximize", "Maximized" {
            w254 = T1."Maximized" ("State")
            n95 = property class="VI"(reference=w260, error in=w259) -> (reference out=w257:refnum<vi>, error out=w258:errorcluster, "FP.State"=w256:T1)
            n96 = Not Equal?(x=w256, y=w254) -> (x != y?=w255:bool)
            n97 = case shown="True" w255 {
              tunnel: [w265 w266] -> w261
              tunnel: w258 -> [w264 w266]
              tunnel: w257 -> [w263 _]
              tunnel: w254 -> [w262 _]
              frame True {
                n98 = invoke class="VI" method="FP.Open"(reference=w263, error in=w264, "State"=w262) -> (error out=w265:errorcluster)  [unwired: 2 in, 4 out]
              }
              frame False {
              }
            }
          }
        }
        n99 = call <vilib>:"Add State(s) to Queue__JKI_lib_State_Machine.vi"("State(s) in (\"\")"=w201) -> ("States Out"=w200:string)  [unwired: 14 in]
      }
      frame "UI: Autoset Arguments" {
        n100 = call "CSM - Revert Arguments-Safe String.vi"("Safe Argument String"=w275) -> ("Origin Argument String"=w267:string)  [unwired: 8 in]
        n101 = control-ref of="CSM"() -> (w270:refnum<vi>)
        n102 = call "Remove Comments from Single-line.vi"("single-line text"=w267) -> ("single-line text without comments"=w274:string)  [unwired: 2 in]
        n103 = call "Split Single-line Message.vi"("single-line text"=w274) -> ("state"=w272:string, "args"=w271:string, "source/target"=w269:string)  [unwired: 6 in, 1 out]
        n104 = case shown="\"<interrupt>\", \"<status>\"" w269 {
          selector: w269 -> [w278 _]
          tunnel: [w278 w279] -> w268
          tunnel: w267 -> [_ w280]
          frame Default {
            (unwired) enum32{"Message", "Status"}."Message" ("Tab(Msg/Status)")
          }
          frame "<interrupt>", "<status>" {
            (unwired) enum32{"Message", "Status"}."Status" ("Tab(Msg/Status)")
            n105 = Match Pattern(string=w280, regular expression="//") -> (after substring=w279:string)  [unwired: 1 in, 3 out]
          }
        }
        n106 = local write "MsgString"(w272) -> ()
        n107 = local write "Arguments"(w271) -> ()
        n108 = property on="Property Node" class="Str"(reference=w270, "Value"=w268) -> ()  [unwired: 1 in, 2 out]
      }
      frame "UI: Refresh History List" {
      }
      frame "CSM: Module Selected" {
        n109 = local write "CSM"(w288) -> ()
        n110 = call <vilib>:"Add State(s) to Queue__jki_lib_state_machine.vi"("State(s) in Front (\"\")"="Action: Refresh API List" ("State(s) in Front (\"\")"), "State(s) in (\"\")"=w286) -> ("States Out"=w287:string)  [unwired: 13 in]
      }
      frame "UI: Refresh UI" {
      }
      frame "---------- Macro ----------" {
        # "Do not put any code in this frame.\n(It is a separator no-op. You can make a copy of this frame to create a new Macro frame)"
        n111 = call <vilib>:"Add State(s) to Queue__JKI_lib_State_Machine.vi"("State(s) in (\"\")"=w297) -> ("States Out"=w296:string)  [unwired: 14 in]
      }
      frame "Macro: Initialize" {
        # "Initialization Macro\n(This is called once, when the VI starts)"
        n112 = call <vilib>:"Add State(s) to Queue__JKI_lib_State_Machine.vi"("State(s) in Front (\"\")"="Data: Initialize\nData: Initialize References\nInitialize Core Data\nUI: Initialize\nData: Load Arguments Config File\nUI: Front Panel State >> Open\nAction: Refresh API List\nAction: Change Btn States", "State(s) in (\"\")"=w302) -> ("States Out"=w301:string)  [unwired: 13 in]
      }
      frame "Macro: Exit" {
        # "Exit Macro\n(This is called once, when the VI exits)"
        n113 = call "FGV-JKISM Modules.vi"("Enum"=_action."Broadcast", "Message"="Macro: Exit") -> ()  [unwired: 8 in, 2 out]
        n114 = call <vilib>:"Add State(s) to Queue__JKI_lib_State_Machine.vi"("State(s) at Back (\"\")"="Data: Save Arguments Config File\nData: Cleanup\nExit") -> ("States Out"=w305:string)  [unwired: 14 in]
        n115 = call <vilib>:"Add State(s) to Queue__JKI_lib_State_Machine.vi"("State(s) in Front (\"\")"=w305, "State(s) in (\"\")"=w310) -> ("States Out"=w309:string)  [unwired: 13 in]
      }
      frame "---------- Action ----------" {
        # "Template Separator\n(You can make a copy of, or modify, this frame)"
        n116 = call <vilib>:"Add State(s) to Queue__JKI_lib_State_Machine.vi"("State(s) in (\"\")"=w314) -> ("States Out"=w313:string)  [unwired: 14 in]
      }
      frame "Action: Send CSM Message" {
        n117 = local read "CSM"() -> (w319:string)
        n118 = Multiply(x=1000, y="Timeout(s)") -> (x*y=w316:i32)
        n119 = case shown="\"\"" "MsgString" {
          selector: "MsgString" -> [_ w332]
          tunnel: "Arguments" -> [_ w331]
          tunnel: [_ w337] -> w320
          tunnel: w319 -> [_ w330]
          tunnel: [_ w329] -> w318
          tunnel: w316 -> [_ w336]
          frame "" {
          }
          frame Default {
            n120 = call "CSM - Send Message and Wait for Reply.vi"("Response Timeout (-2 Using Global Settings)"=w336, "Current Module (\"\" to Generate an ID)"="Tool-Testpnl" ("Current Module(\"\" to generate an ID)"), "Target Module"=w330, "Arguments (\"\")"=w331, "State"=w332) -> ("error out"=w337:errorcluster, "Response"=w339:string)  [unwired: 4 in, 1 out]
            n121 = call-poly "Build Message with Arguments++.vi"("State With Arguments"=w332, "Arguments (\"\")"=w331, "Target Module (\"\")"=w330) -> ("CSM Message String"=w334:string)  [unwired: 12 in]
            n122 = case shown="True" "Revert Safe String" {
              tunnel: w339 -> [w340 w342]
              tunnel: [w340 w341] -> w327
              frame False {
              }
              frame True {
                n123 = call "CSM - Revert Arguments-Safe String.vi"("Safe Argument String"=w342) -> ("Origin Argument String"=w341:string)  [unwired: 8 in]
              }
            }
            "Response" <- w327
            n124 = call "CSM - Make String Arguments Safe.vi"("Argument String"=w334) -> ("Safe Argument String"=w333:string)  [unwired: 8 in]
            n125 = call <vilib>:"Build State String with Arguments__JKI_lib_State_Machine.vi"("Arguments (\"\")"=w333, "State"="" ("State(s) in Front (\"\")")) -> ("State with Arguments"=w328:string)  [unwired: 4 in]
            n126 = call <vilib>:"Add State(s) to Queue__JKI_lib_State_Machine.vi"("State(s) in (\"\")"=w328) -> ("States Out"=w329:string)  [unwired: 14 in]
          }
        }
        n127 = call <vilib>:"Add State(s) to Queue__JKI_lib_State_Machine.vi"("State(s) in (\"\")"=w325, "State(s) at Back (\"\")"=w318) -> ("States Out"=w324:string)  [unwired: 13 in]
      }
      frame "Action: Post CSM Message" {
        # "Your code here.\n(You can make a copy of, or modify, this frame)"
        n128 = local read "MsgString"() -> (w343:string)
        n129 = local read "Arguments"() -> (w344:string)
        n130 = local read "CSM"() -> (w346:string)
        n131 = case shown="Default" w343 {
          selector: w343 -> [_ w356]
          tunnel: w344 -> [_ w355]
          tunnel: [_ w360] -> w347
          tunnel: w346 -> [_ w354]
          tunnel: [_ w353] -> w345
          frame "" {
          }
          frame Default {
            n132 = call "CSM - Post Message.vi"("Current Module (\"\" to Generate an ID)"="Tool-Testpnl" ("Current Module(\"\" to generate an ID)"), "Target Module"=w354, "Arguments (\"\")"=w355, "State"=w356) -> ("error out"=w360:errorcluster)  [unwired: 7 in]
            n133 = call-poly "Build Message with Arguments++.vi"("State With Arguments"=w356, "Arguments (\"\")"=w355, "Target Module (\"\")"=w354) -> ("CSM Message String"=w358:string)  [unwired: 12 in]
            n134 = call "CSM - Make String Arguments Safe.vi"("Argument String"=w358) -> ("Safe Argument String"=w357:string)  [unwired: 8 in]
            n135 = call <vilib>:"Build State String with Arguments__JKI_lib_State_Machine.vi"("Arguments (\"\")"=w357, "State"="" ("State(s) in Front (\"\")")) -> ("State with Arguments"=w352:string)  [unwired: 4 in]
            n136 = call <vilib>:"Add State(s) to Queue__JKI_lib_State_Machine.vi"("State(s) in (\"\")"=w352, "State(s) at Back (\"\")"="UI: Refresh History List\nData: Save Arguments Config File" ("State(s) in Front (\"\")")) -> ("States Out"=w353:string)  [unwired: 13 in]
          }
        }
        n137 = call <vilib>:"Add State(s) to Queue__JKI_lib_State_Machine.vi"("State(s) in (\"\")"=w350, "State(s) at Back (\"\")"=w345) -> ("States Out"=w349:string)  [unwired: 13 in]
      }
      frame "Action: Broadcast Status" {
        # "Your code here.\n(You can make a copy of, or modify, this frame)"
        n138 = local read "MsgString"() -> (w362:string)
        n139 = local read "Arguments"() -> (w363:string)
        n140 = local read "CSM"() -> (w365:string)
        n141 = case shown="Default" w362 {
          selector: w362 -> [_ w372]
          tunnel: w363 -> [_ w371]
          tunnel: [_ w373] -> w366
          tunnel: w365 -> [_ w370]
          tunnel: [_ w378] -> w364
          frame "" {
          }
          frame Default {
            (unwired) "Tool-Testpnl" ("Current Module(\"\" to generate an ID)")
            n142 = call "CSM - Request CSM to Broadcast Status Change.vi"("Module Name"=w370, "Arguments (\"\")"=w371, "Status"=w372) -> ("error out"=w373:errorcluster)  [unwired: 8 in]
            n143 = call-poly "Build Message with Arguments++.vi"("State With Arguments"=w372, "Arguments (\"\")"=w371) -> ("CSM Message String"=w380:string)  [unwired: 13 in]
            n144 = Concatenate Strings(w380, "//" ("string"), w370) -> (w375:string)
            n145 = call "CSM - Make String Arguments Safe.vi"("Argument String"=w375) -> ("Safe Argument String"=w379:string)  [unwired: 8 in]
            n146 = call <vilib>:"Build State String with Arguments__JKI_lib_State_Machine.vi"("Arguments (\"\")"=w379, "State"="" ("State(s) in Front (\"\")")) -> ("State with Arguments"=w377:string)  [unwired: 4 in]
            n147 = call <vilib>:"Add State(s) to Queue__JKI_lib_State_Machine.vi"("State(s) in (\"\")"=w377, "State(s) at Back (\"\")"="UI: Refresh History List\nData: Save Arguments Config File" ("State(s) in Front (\"\")")) -> ("States Out"=w378:string)  [unwired: 13 in]
          }
        }
        n148 = call <vilib>:"Add State(s) to Queue__JKI_lib_State_Machine.vi"("State(s) in (\"\")"=w369, "State(s) at Back (\"\")"=w364) -> ("States Out"=w368:string)  [unwired: 13 in]
      }
      frame "Action: Change Btn States" {
      }
      frame "Action: Refresh API List" {
        n149 = local read "CSM"() -> (w389:string)
        n150 = in-place {
          in-place-border: w389 -> [w400]
          in-place-border: [w399] -> w392
          n151 = in-place-cluster #1(w391) -> ("CSM Check History"=w398:string[])
          n152 = Search 1D Array(1D array=w398, element=w400) -> (index of element=w401:i32)  [unwired: 1 in]
          n153 = Less Than 0?(x=w401) -> (x < 0?=w399:bool)
          n154 = case shown="True" w399 {
            tunnel: w398 -> [w402 w405]
            tunnel: w400 -> [_ w404]
            tunnel: [w402 w403] -> w397
            frame False {
            }
            frame True {
              n155 = Build Array (concatenate)(w405, w404) -> (w403:string[])
            }
          }
          n156 = in-place-cluster #1("CSM Check History"=w397) -> (w390:T6)
        }
        n157 = call "CSM - Check If Module Exists.vi"("CSM Name"=w389) -> ("error out"=w386:errorcluster, "Exist?"=w387:bool, "CSM Name (Dup)"=w395:string)  [unwired: 8 in]
        n158 = Not(x=w386) -> (.not. x?=w385:bool)
        n159 = And(x=w387, y=w385) -> (x .and. y?=w388:bool)
        n160 = case shown="False" w388 {
          tunnel: w395 -> [_ w421]
          tunnel: w394 -> [_ w420]
          tunnel: [_ w422] -> w393
          tunnel: w392 -> [_ w419]
          frame False {
            w407 = T8."Disabled and Grayed Out" ("Disabled")
            n161 = property on="Message/Status" class="CmbBox"("Strings[]"=string[] [] ("Strings []")) -> ()  [unwired: 2 in, 2 out]
            n162 = property on="Revert Safe String" class="Bool (strict)"("DisabledEnum"=w407) -> ()  [unwired: 2 in, 2 out]
            n163 = property on="Arguments" class="Str"("DisabledEnum"=w407) -> ()  [unwired: 2 in, 2 out]
            n164 = property on="Response" class="Str"("DisabledEnum"=w407) -> ()  [unwired: 2 in, 2 out]
          }
          frame True {
            w414 = T8."Enabled" ("Disabled")
            n165 = call "Read CSM States with lvcsm Support.vi"("Current Module (\"\" to Generate an ID)"=w420, "Force? (F)"=w419, "CSM Name"=w421) -> ("error out"=w422:errorcluster, "CSMAPI List"=w409:string[])  [unwired: 7 in]
            n166 = call "filter CSM States.vi"("Interface-Filter"="Interface-Filter", "Array"=w409) -> ("filtered array"=w416:string[])  [unwired: 9 in]
            n167 = property on="Revert Safe String" class="Bool (strict)"("DisabledEnum"=w414) -> ()  [unwired: 2 in, 2 out]
            n168 = property on="Arguments" class="Str"("DisabledEnum"=w414) -> ()  [unwired: 2 in, 2 out]
            n169 = property on="Response" class="Str"("DisabledEnum"=w414) -> ()  [unwired: 2 in, 2 out]
            n170 = property on="Message/Status" class="CmbBox"("Strings[]"=w416) -> ("Value"=w417:string)  [unwired: 2 in, 2 out]
            n171 = Search 1D Array(1D array=w416, element=w417) -> (index of element=w418:i32)  [unwired: 1 in]
            n172 = Index Array(array=w416) -> (element=w411:string)  [unwired: 1 in]
            n173 = Greater Or Equal To 0?(x=w418) -> (x >= 0?=w412:bool)
            n174 = Empty String/Path?(string/path=w411) -> (empty?=w410:bool)
            n175 = Or(x=w412, y=w410) -> (x .or. y?=w413:bool)
            n176 = Select(t=w417, s=w413, f=w411) -> (s? t:f=w415:string)
            n177 = property on="Message/Status" class="CmbBox"("Value"=w415) -> ()  [unwired: 2 in, 2 out]
          }
        }
      }
      frame "No Peroidic Log over 1s" {
      }
    }
  }
  n178 = disable-structure shown="Disabled" {
    frame Disabled {
      n179 = case shown="\"Module Created\", \"Module Destroyed\"" {
        selector: _ -> [_ _]
        tunnel: _ -> [_ w427]
        frame "User Log", Default {
        }
        frame "Module Created", "Module Destroyed" {
          n180 = Generate User Event(user event=w427, event data cluster="UI: Refresh CSM List" ("State(s) in Front (\"\")")) -> ()  [unwired: 2 in, 2 out]
        }
      }
    }
    frame Enabled {
    }
  }
  n181 = control-ref of="Current VI Reference"() -> (w4:refnum<vi>)
  n182 = call "Close FP if in LabVIEW Dir.vi"("VI Refnum"=w4, "Error in"=w3) -> ("Error out"=w5:errorcluster)  [unwired: 9 in]
  n183 = call <vilib>:"Clear Errors.vi"("error in (no error)"=w5) -> ()  [unwired: 5 in, 2 out]
